vi "VRM_to_DSC.vi"(4 "error in (no error)":errorcluster, 5 "VRM Actions":T1, 7 "VRM status":T2={"X Target (T)"=0.0, "Y Target (T)"=0.0, "Z Target (T)"=0.0, "X Field (T)"=-0.0, "Y Field (T)"=0.0, "Z Field (T)"=0.0, "X Rate (T/min)"=0.0002, "Y Rate (T/min)"=0.0002, "Z Rate (T/min)"=0.05, "X Current (A)"=-0.0001, "Y Current (A)"=0.0001, "Z Current (A)"=0.0, "X Voltage (V)"=0.0003, "Y Voltage (V)"=0.0, "Z Voltage (V)"=-0.0001}) -> (0 "error out":errorcluster)   [LabVIEW 2016]
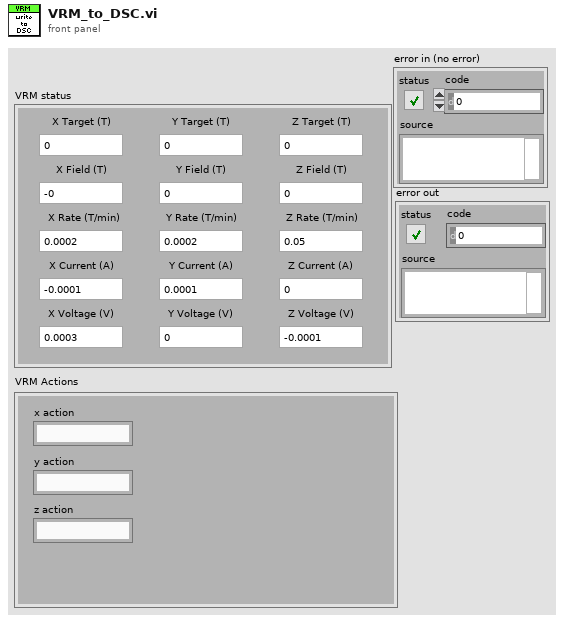
[diagram p1: front panel]
types:
  T1 = cluster{"x action":string, "y action":string, "z action":string}
  T2 = cluster{"X Target (T)":dbl, "Y Target (T)":dbl, "Z Target (T)":dbl, "X Field (T)":dbl, "Y Field (T)":dbl, "Z Field (T)":dbl, "X Rate (T/min)":dbl, "Y Rate (T/min)":dbl, "Z Rate (T/min)":dbl, "X Current (A)":dbl, "Y Current (A)":dbl, "Z Current (A)":dbl, "X Voltage (V)":dbl, "Y Voltage (V)":dbl, "Z Voltage (V)":dbl}
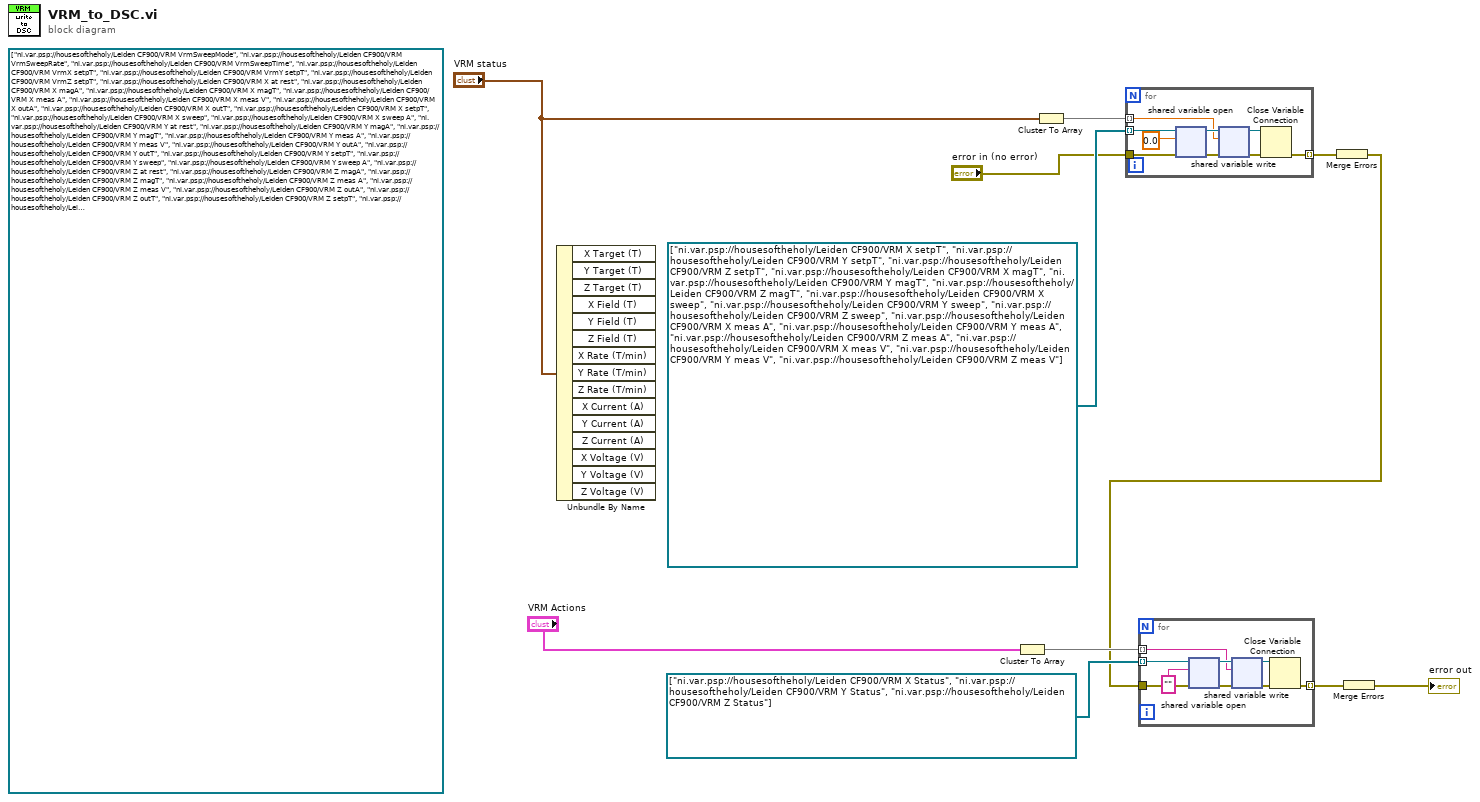
[diagram p0: block diagram]
diagram:
  (unwired) refnum<k21>[] ["ni.var.psp://housesoftheholy/Leiden CF900/VRM VrmSweepMode", "ni.var.psp://housesoftheholy/Leiden CF900/VRM VrmSweepRate", "ni.var.psp://housesoftheholy/Leiden CF900/VRM VrmSweepTime", "ni.var.psp://housesoftheholy/Leiden CF900/VRM VrmX setpT", "ni.var.psp://housesoftheholy/Leiden CF900/VRM VrmY setpT", "ni.var.psp://housesoftheholy/Leiden CF900/VRM VrmZ setpT", "ni.var.psp://housesoftheholy/Leiden CF900/VRM X at rest", "ni.var.psp://housesoftheholy/Leiden CF900/VRM X magA", "ni.var.psp://housesoftheholy/Leiden CF900/VRM X magT", "ni.var.psp://housesoftheholy/Leiden CF900/VRM X meas A", "ni.var.psp://housesoftheholy/Leiden CF900/VRM X meas V", "ni.var.psp://housesoftheholy/Leiden CF900/VRM X outA", "ni.var.psp://housesoftheholy/Leiden CF900/VRM X outT", "ni.var.psp://housesoftheholy/Leiden CF900/VRM X setpT", "ni.var.psp://housesoftheholy/Leiden CF900/VRM X sweep", "ni.var.psp://housesoftheholy/Leiden CF900/VRM X sweep A", "ni.var.psp://housesoftheholy/Leiden CF900/VRM Y at rest", "ni.var.psp://housesoftheholy/Leiden CF900/VRM Y magA", "ni.var.psp://housesoftheholy/Leiden CF900/VRM Y magT", "ni.var.psp://housesoftheholy/Leiden CF900/VRM Y meas A", "ni.var.psp://housesoftheholy/Leiden CF900/VRM Y meas V", "ni.var.psp://housesoftheholy/Leiden CF900/VRM Y outA", "ni.var.psp://housesoftheholy/Leiden CF900/VRM Y outT", "ni.var.psp://housesoftheholy/Leiden CF900/VRM Y setpT", "ni.var.psp://housesoftheholy/Leiden CF900/VRM Y sweep", "ni.var.psp://housesoftheholy/Leiden CF900/VRM Y sweep A", "ni.var.psp://housesoftheholy/Leiden CF900/VRM Z at rest", "ni.var.psp://housesoftheholy/Leiden CF900/VRM Z magA", "ni.var.psp://housesoftheholy/Leiden CF900/VRM Z magT", "ni.var.psp://housesoftheholy/Leiden CF900/VRM Z meas A", "ni.var.psp://housesoftheholy/Leiden CF900/VRM Z meas V", "ni.var.psp://housesoftheholy/Leiden CF900/VRM Z outA", "ni.var.psp://housesoftheholy/Leiden CF900/VRM Z outT", "ni.var.psp://housesoftheholy/Leiden CF900/VRM Z setpT", "ni.var.psp://housesoftheholy/Leiden CF900/VRM Z sweep", "ni.var.psp://housesoftheholy/Leiden CF900/VRM Z sweep A"]
  n1 = Unbundle By Name("VRM status") -> ()  [unwired: 15 out]
  n2 = Cluster To Array(cluster="VRM Actions") -> (array=w7:string[])
  n3 = Cluster To Array(cluster="VRM status") -> (array=w11:dbl[])
  n4 = for {
    tunnel: refnum<k21>[] ["ni.var.psp://housesoftheholy/Leiden CF900/VRM X setpT", "ni.var.psp://housesoftheholy/Leiden CF900/VRM Y setpT", "ni.var.psp://housesoftheholy/Leiden CF900/VRM Z setpT", "ni.var.psp://housesoftheholy/Leiden CF900/VRM X magT", "ni.var.psp://housesoftheholy/Leiden CF900/VRM Y magT", "ni.var.psp://housesoftheholy/Leiden CF900/VRM Z magT", "ni.var.psp://housesoftheholy/Leiden CF900/VRM X sweep", "ni.var.psp://housesoftheholy/Leiden CF900/VRM Y sweep", "ni.var.psp://housesoftheholy/Leiden CF900/VRM Z sweep", "ni.var.psp://housesoftheholy/Leiden CF900/VRM X meas A", "ni.var.psp://housesoftheholy/Leiden CF900/VRM Y meas A", "ni.var.psp://housesoftheholy/Leiden CF900/VRM Z meas A", "ni.var.psp://housesoftheholy/Leiden CF900/VRM X meas V", "ni.var.psp://housesoftheholy/Leiden CF900/VRM Y meas V", "ni.var.psp://housesoftheholy/Leiden CF900/VRM Z meas V"] -> [w16] mode=indexing
    tunnel: w11 -> [w15] mode=indexing
    tunnel: [w13] -> w4 mode=indexing
    tunnel: "error in (no error)" -> [w12]
    n5 = shared-variable-open(w16, w12, 0.0) -> (w19:refnum<k21>, w18:errorcluster)  [unwired: 1 in]
    n6 = shared-variable-write(w19, w18, w15) -> (w20:refnum<k21>, w17:errorcluster)
    n7 = Close Variable Connection(8:w17, 11:w20) -> (0:w13:errorcluster)
  }
  n8 = Merge Errors(w4) -> (w3:errorcluster)
  n9 = for {
    tunnel: refnum<k21>[] ["ni.var.psp://housesoftheholy/Leiden CF900/VRM X Status", "ni.var.psp://housesoftheholy/Leiden CF900/VRM Y Status", "ni.var.psp://housesoftheholy/Leiden CF900/VRM Z Status"] -> [w25] mode=indexing
    tunnel: w7 -> [w24] mode=indexing
    tunnel: [w22] -> w2 mode=indexing
    tunnel: w3 -> [w21]
    n10 = shared-variable-open(w25, w21, "") -> (w28:refnum<k21>, w27:errorcluster)  [unwired: 1 in]
    n11 = shared-variable-write(w28, w27, w24) -> (w29:refnum<k21>, w26:errorcluster)
    n12 = Close Variable Connection(8:w26, 11:w29) -> (0:w22:errorcluster)
  }
  n13 = Merge Errors(w2) -> (→"error out":errorcluster)
